vi "PH_AxisGUI_BaseClass.PC Set Zero.vi"(0 "VI in":refnum<vi>, 2 "Axis":i32=-1, 5 "error in (no error)":errorcluster) -> (14 "VI out":refnum<vi>, 19 "error out":errorcluster)   [LabVIEW 2014, in "PH_AxisGUI_BaseClass.lvlib"]
doc: "This VI acts on an axis."
uses:
  PH_AxisGUI_BaseClass.lvlib
  PH_Stepmotor_BaseClass/PH_Stepmotor_BaseClass.lvlib
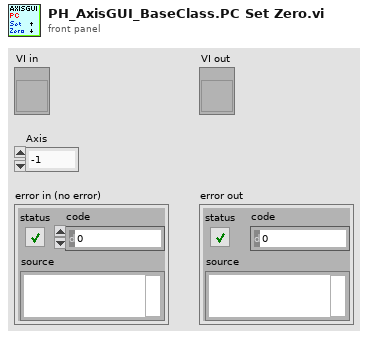
[diagram p1: front panel]
types:
  T1 = typedef "PH_Stepmotor_BaseClass.lvlib/PH_Stepmotor_BaseClass.Axis Address.ctl" = cluster{"Instance":string, "Motor Nr":i32}
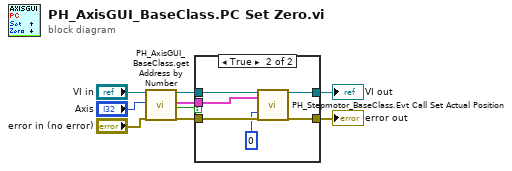
[diagram p0: block diagram]
diagram:
  n1 = call "PH_AxisGUI_BaseClass.get Address by Number.vi"("VI in"="VI in", "Axis"="Axis", "error in (no error)"="error in (no error)") -> ("VI out"=w9:refnum<vi>, "Address"=w3:T1, "Axis exists and is not moving?"=w2:bool, "error out"=w7:errorcluster)  [unwired: 12 in, 1 out]
  n2 = case shown="True" w2 {
    tunnel: [w11 w12] -> w5
    tunnel: [w10 w13] -> w6
    tunnel: w7 -> [w10 w17]
    tunnel: w9 -> [w11 w16]
    tunnel: w3 -> [_ w15]
    frame False {
    }
    frame True {
      n3 = call "PH_Stepmotor_BaseClass.Evt Call Set Actual Position.vi"("i ref in"=w16, "Address"=w15, "Position to set [Steps]"=0 ("Define Position"), "error in"=w17) -> ("i ref out"=w12:refnum<vi>, "error out"=w13:errorcluster)  [unwired: 14 in]
    }
  }
  "error out" <- w6
  "VI out" <- w5
